vi "Shift coordinates (IMAQ to SLM).vi"(5 "Trap cluster":T1, 7 "Coordinate mapping \n(IMAQ to SLM)":T2) -> (0 "X (SLM)":dbl[](array[numeric]), 1 "Y (SLM)":dbl[](array[numeric]), 2 "Amplitudes":dbl[](array[numeric]), 3 "Number of traps":i32, 4 "Z (SLM)":dbl[](array[numeric]))   [LabVIEW 8.6]
uses:
  Trap cluster.ctl
panel:
  out "element":T1
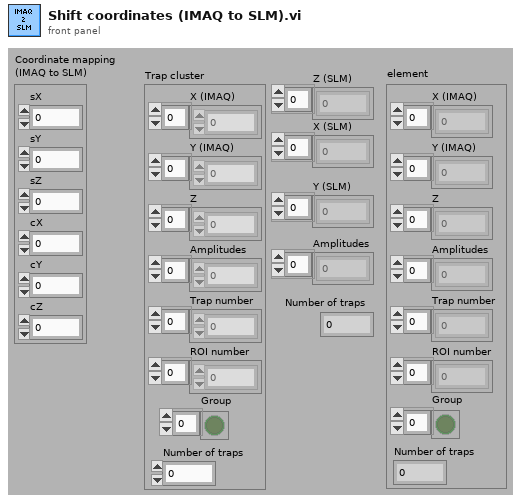
[diagram p1: front panel]
types:
  T1 = typedef "Trap cluster.ctl" = cluster{"X (IMAQ)":dbl[], "Y (IMAQ)":dbl[], "Z":dbl[], "Amplitudes":dbl[], "Trap number":i32[], "ROI number":i32[], "Number of traps":i32, "Group":bool[]}
  T2 = cluster{"sX":dbl, "sY":dbl, "sZ":dbl, "cX":dbl, "cY":dbl, "cZ":dbl}
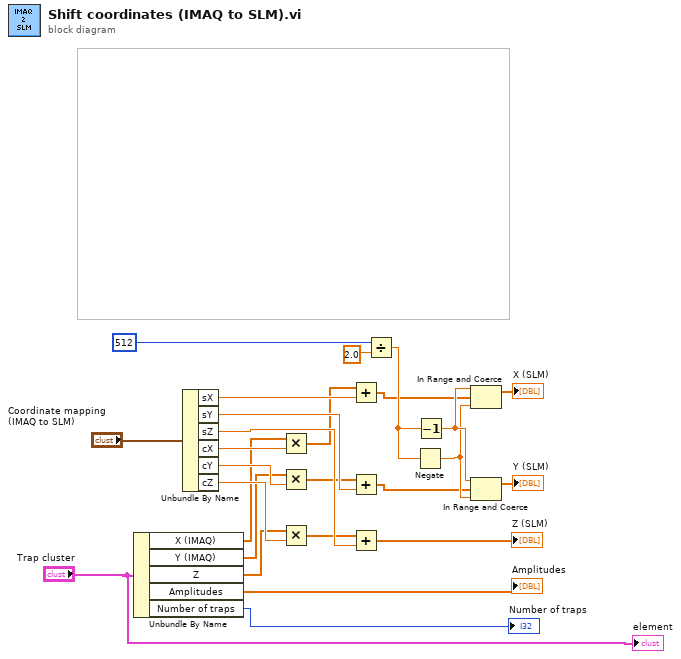
[diagram p0: block diagram]
diagram:
  n1 = Unbundle By Name("Trap cluster") -> ("X (IMAQ)"=w11:dbl[], "Y (IMAQ)"=w10:dbl[], "Z"=w9:dbl[], "Amplitudes"=→"Amplitudes":dbl[], "Number of traps"=→"Number of traps":i32)
  n2 = Unbundle By Name("Coordinate mapping \n(IMAQ to SLM)") -> ("sX"=w21:dbl, "sY"=w22:dbl, "sZ"=w23:dbl, "cX"=w24:dbl, "cY"=w25:dbl, "cZ"=w26:dbl)
  n3 = Multiply(x=w11, y=w24) -> (x*y=w16:dbl[])
  n4 = Multiply(x=w10, y=w25) -> (x*y=w17:dbl[])
  n5 = Multiply(x=w9, y=w26) -> (x*y=w18:dbl[])
  n6 = Add(x=w16, y=w21) -> (x+y=w2:dbl[])
  n7 = Add(x=w17, y=w22) -> (x+y=w1:dbl[])
  n8 = Add(x=w18, y=w23) -> (x+y=→"Z (SLM)":dbl[])
  n9 = Divide(x=512 ("SLM size"), y=2.0) -> (x/y=w4:dbl)
  n10 = Negate(x=w4) -> (-x=w3:dbl)
  n11 = Decrement(x=w4) -> (x-1=w5:dbl)
  n12 = In Range and Coerce(upper limit=w5, x=w2, lower limit=w3) -> (coerced(x)=→"X (SLM)":dbl[])  [unwired: 1 out]
  n13 = In Range and Coerce(upper limit=w5, x=w1, lower limit=w3) -> (coerced(x)=→"Y (SLM)":dbl[])  [unwired: 1 out]
  "element" <- "Trap cluster"
